vi "AreaPerimeterCalculationMG.vi"() -> ()   [LabVIEW 2012]
doc: "This VI uses a given radius/side length to calculate the area/perimeter of a circle/square. The user gets to choose what they want to calculate and for what shape"
panel:
  in  "Area of Perimeter of S":u16(ring) items=["Perimeter", "Area"]
  out "SO":dbl
  in  "SI":dbl
  out "CO":dbl
  in  "Area or Perimeter of C":u16(ring) items=["Perimeter", "Area"]
  in  "CI":dbl
  # "Marco Gonzalez\nEA3\n02 / 28 /2017"
  # "Circle"
  # "Square"
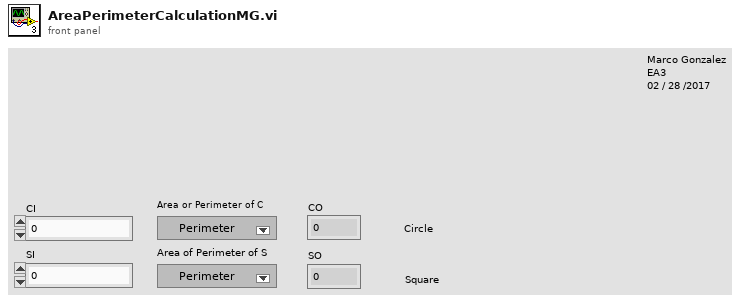
[diagram p1: front panel]
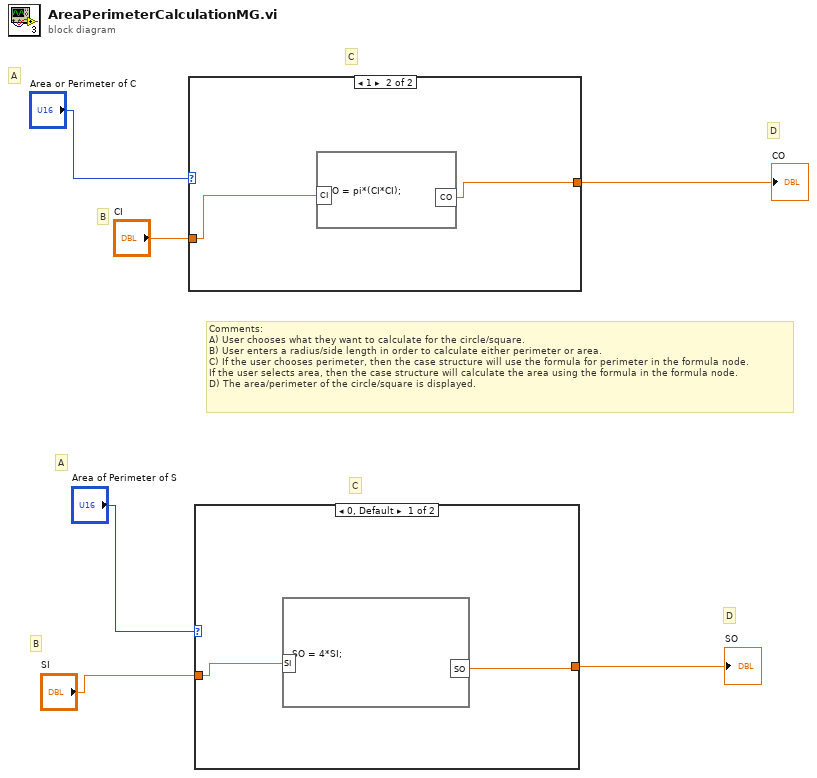
[diagram p0: block diagram]
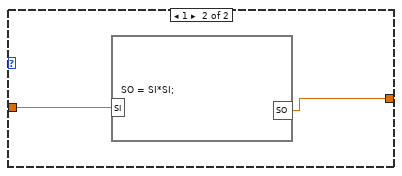
[diagram p2: hidden frame]
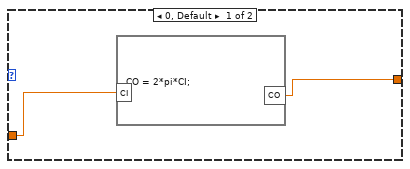
[diagram p3: hidden frame]
diagram:
  # "D"
  # "D"
  # "C"
  # "C"
  # "B"
  # "B"
  # "Comments:\nA) User chooses what they want to calculate for the circle/square.\nB) User enters a radius/side length in order to calculate either perimeter or area.\nC) If the user chooses perimeter, then the case structure will use the formula for perimeter in the formula node.\nIf the user selects area, then the case structure will calculate the area using the formula in the formula node.\nD) The area/perimeter of the circle/square is displayed."
  # "A"
  # "A"
  n1 = case shown="1" "Area or Perimeter of C" {
    tunnel: "CI" -> [w8 w10]
    tunnel: [w7 w9] -> w4
    frame 0, Default {
      n2 = formula code="CO = 2*pi*CI;"("CI"=w8) -> ("CO"=w7:dbl)
    }
    frame 1 {
      n3 = formula code="CO = pi*(CI*CI);"("CI"=w10) -> ("CO"=w9:dbl)
    }
  }
  "CO" <- w4
  n4 = case shown="0, Default" "Area of Perimeter of S" {
    tunnel: "SI" -> [w12 w14]
    tunnel: [w11 w13] -> w1
    frame 0, Default {
      n5 = formula code="SO = 4*SI;"("SI"=w12) -> ("SO"=w11:dbl)
    }
    frame 1 {
      n6 = formula code="SO = SI*SI;"("SI"=w14) -> ("SO"=w13:dbl)
    }
  }
  "SO" <- w1
